vi "Example 4.vi"() -> ()   [LabVIEW 2018]
uses:
  <vilib>/addons/VeriStand Custom Device Scripting APIs/FPGA Addon/Scripting API.lvlib
panel:
  out "error out":errorcluster
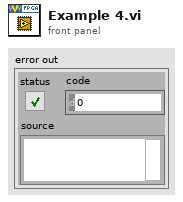
[diagram p1: front panel]
types:
  T1 = typedef "Custom Device API.lvlib/Custom Device Item Ref.ctl" = u64
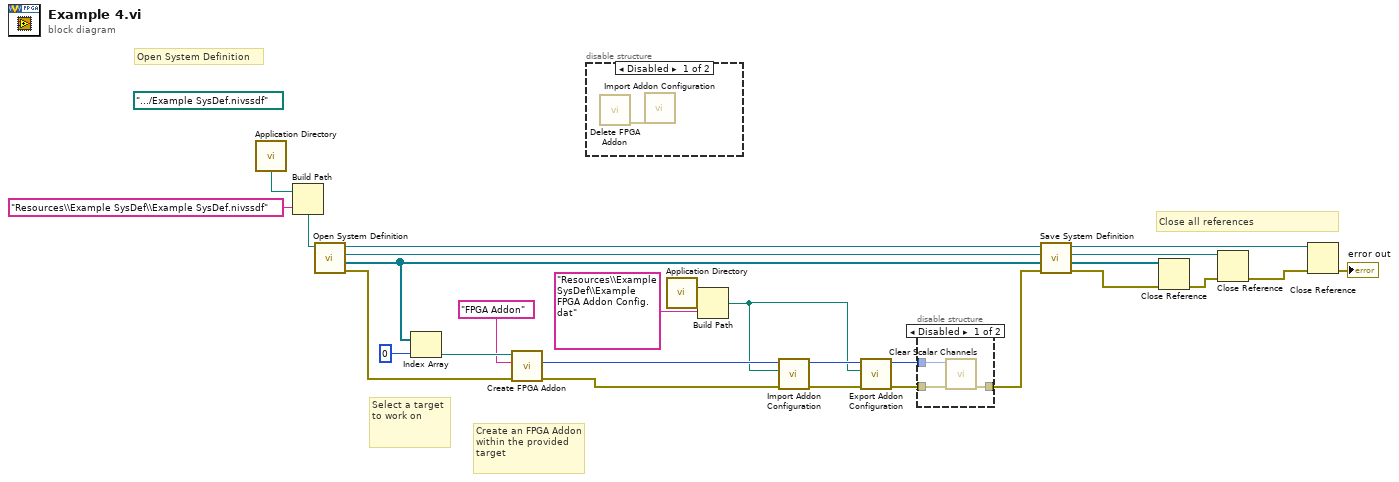
[diagram p0: block diagram]
diagram:
  (unwired) path ".../Example SysDef.nivssdf" ("fpga bitfile path")
  # "Close all references"
  # "Create an FPGA Addon within the provided target"
  # "Select a target to work on"
  # "Open System Definition"
  n1 = call <vilib>:"Application Directory.vi"() -> ("Application Directory"=w17:path)
  n2 = Build Path(base path=w17, name or relative path="Resources\\Example SysDef\\Example SysDef.nivssdf") -> (appended path=w15:path)
  n3 = call "Open System Definition.vi"("System Definition File"=w15) -> ("error out"=w22:errorcluster, "targets refnums"=w20:refnum<k24>[], "root refnum"=w21:refnum<k24>, "system definition refnum"=w13:refnum<k24>)  [unwired: 7 in]
  n4 = Index Array(array=w20, index=0) -> (element=w24:refnum<k24>)
  n5 = call <vilib>:"Create FPGA Addon.vi"("error in (no error)"=w22, "FPGA Addon name"="FPGA Addon" ("fpga addon name"), "target in"=w24) -> ("error out"=w10:errorcluster, "FPGA Addon refnum"=w9:T1)  [unwired: 6 in, 1 out]
  n6 = disable-structure shown="Disabled" {
    frame Disabled {
      n7 = call <vilib>:"Delete FPGA Addon.vi"() -> ("error out"=w26:errorcluster)  [unwired: 10 in, 1 out]
      n8 = call <vilib>:"Import Addon Configuration.vi"("error in (no error)"=w26) -> ()  [unwired: 9 in, 2 out]
    }
    frame Enabled {
    }
  }
  n9 = call <vilib>:"Application Directory.vi"() -> ("Application Directory"=w7:path)
  n10 = Build Path(base path=w7, name or relative path="Resources\\Example SysDef\\Example FPGA Addon Config.dat") -> (appended path=w4:path)
  n11 = call <vilib>:"Import Addon Configuration.vi"("error in (no error)"=w10, "configuration file path"=w4, "FPGA Addon refnum in"=w9) -> ("error out"=w6:errorcluster, "FPGA Addon refnum out"=w5:T1)  [unwired: 7 in]
  n12 = call <vilib>:"Export Addon Configuration.vi"("error in (no error)"=w6, "export file path"=w4, "FPGA Addon refnum in"=w5) -> ("error out"=w3:errorcluster, "FPGA Addon refnum out"=w2:T1)  [unwired: 7 in]
  n13 = disable-structure shown="Disabled" {
    disable-tunnel: w3 -> [w29 w30]
    disable-tunnel: w2 -> [w28 _]
    disable-tunnel: [w27 w30] -> w1
    frame Disabled {
      n14 = call <vilib>:"Clear Scalar Channels.vi"("error in (no error)"=w29, "FPGA Addon refnum in"=w28) -> ("error out"=w27:errorcluster)  [unwired: 8 in, 1 out]
    }
    frame Enabled {
    }
  }
  n15 = call "Save System Definition.vi"("error in (no error)"=w1, ".NET Refnum in"=w13) -> ("error out"=w11:errorcluster, ".NET Refnum out"=w12:refnum<k24>)  [unwired: 8 in]
  n16 = Close Reference(reference=w20, error in (no error)=w11) -> (error out=w19:errorcluster)
  n17 = Close Reference(reference=w21, error in (no error)=w19) -> (error out=w18:errorcluster)
  n18 = Close Reference(reference=w12, error in (no error)=w18) -> (error out=→"error out":errorcluster)
